vi "Is slot empty.vi"(8 "error in (no error)":errorcluster, 10 "Card Position":T1, 11 "Node Ptr":u64 format="%.0x") -> (0 "error out":errorcluster, 1 "Empty?":bool, 3 "Node Ptr out":u64 format="%.0x")   [LabVIEW 2014, in "SLSC configuration System Explorer.lvlib"]
uses:
  SLSC configuration System Explorer.lvlib
  Shared/Card Postion.ctl
  Shared/Constants.vi
  <vilib>/NI Veristand/Custom Device API/Get Item Property (Variant).vi
  <vilib>/NI Veristand/Custom Device API/Custom Device API.lvlib
  Shared/SLSC configuration Shared.lvlib
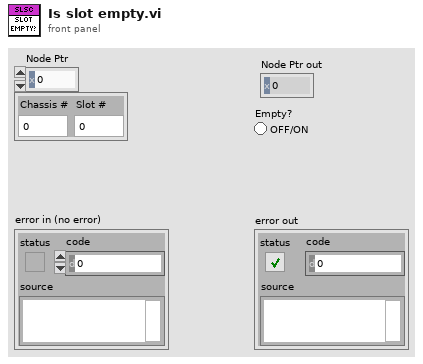
[diagram p1: front panel]
types:
  T1 = typedef "SLSC configuration Shared.lvlib/Card Postion.ctl" = cluster{"Chassis #":u8, "Slot #":u8}
  T2 = typedef "Custom Device API.lvlib/Custom Device Item Ref.ctl" = u64
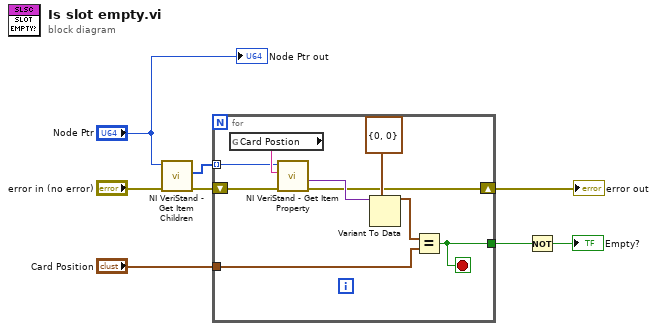
[diagram p0: block diagram]
diagram:
  n1 = call <vilib>:"NI VeriStand - Get Item Children.vi"("error in (no error)"="error in (no error)", "Item Ref in"="Node Ptr") -> ("error out"=w4:errorcluster, "Child Refs"=w2:T2[])  [unwired: 6 in, 2 out]
  n2 = for {
    tunnel: "Card Position" -> [w13]
    tunnel: [w12] -> w7
    shift-right: [w10] -> w3
    shift-left: w4 -> [w11]
    tunnel: w2 -> [w9] mode=indexing
    stop <- w12 stop-if-true
    n3 = global read "Constants.vi" "Card Postion"() -> (w17:string)
    n4 = call-poly <vilib>:"NI VeriStand - Get Item Property.vi"("error in (no error)"=w11, "Property Name"=w17, "Item Ref in"=w9) -> ("error out"=w10:errorcluster, "Value"=w16:variant)  [unwired: 5 in, 2 out]
    n5 = Variant To Data(type=T1 {"Chassis #"=0, "Slot #"=0} ("Card Position"), Variant=w16) -> (data=w14:T1)  [unwired: 1 in, 1 out]
    n6 = Equal?(x=w14, y=w13) -> (x = y?=w12:bool)
  }
  "error out" <- w3
  n7 = Not(x=w7) -> (.not. x?=→"Empty?":bool)
  "Node Ptr out" <- "Node Ptr"
